vi "CANReadBaseTime.vi"(7 "时间":u32, 8 "日期字符":string) -> (2 "基时间簇":T1)   [LabVIEW 2015]
uses:
  <vilib>/Utility/miscctls.llb/LVDateTimeRec.ctl
  <vilib>/regexp/Match Regular Expression.xnode
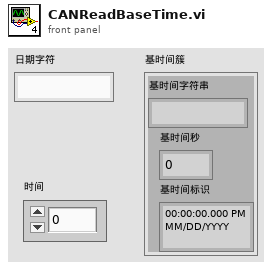
[diagram p1: front panel]
types:
  T1 = cluster{"基时间字符串":string, "基时间秒":dbl, "基时间标识":timestamp}
  T2 = typedef "LVDateTimeRec.ctl" = cluster{"fractional second":dbl, "second":i32, "minute":i32, "hour":i32, "day of month":i32, "month":i32, "year":i32, "day of week":i32, "day of year":i32, "DST":i32}
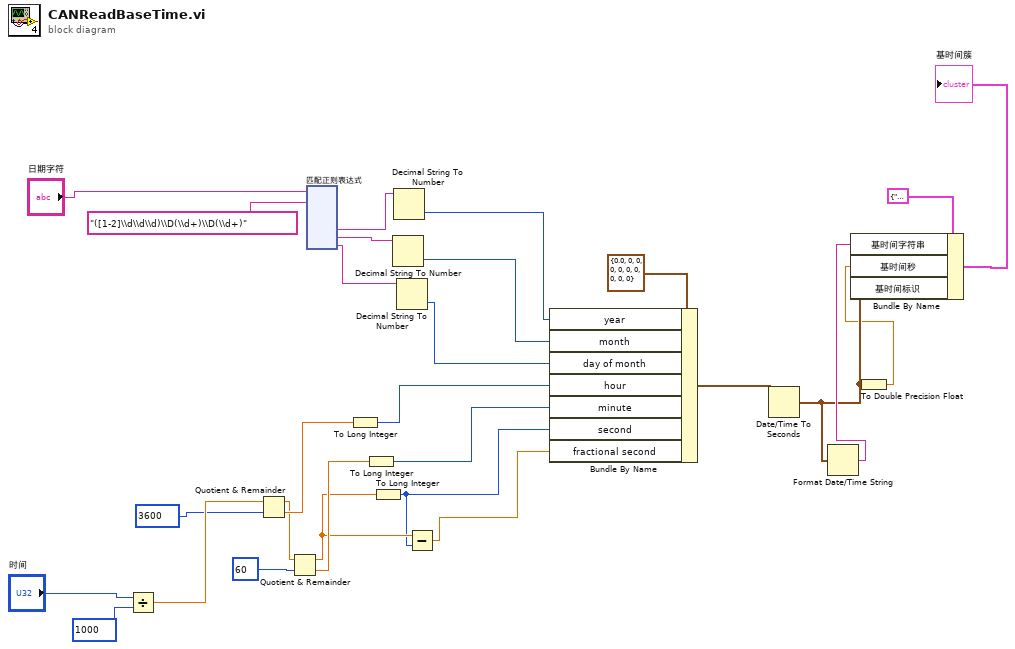
[diagram p0: block diagram]
diagram:
  n1 = Divide(x="时间", y=u32 1000) -> (x/y=w11:dbl)
  n2 = Quotient & Remainder(x=w11, y=3600) -> (x-y*floor(x/y)=w6:dbl, floor(x/y)=w9:dbl)
  n3 = Quotient & Remainder(x=w6, y=60) -> (x-y*floor(x/y)=w3:dbl, floor(x/y)=w5:dbl)
  n4 = xnode "匹配正则表达式"("输入字符串"="日期字符", "正则表达式"="([1-2]\\d\\d\\d)\\D(\\d+)\\D(\\d+)") -> ("子匹配 1"=w20:string, "子匹配 2"=w19:string, "子匹配 3"=w18:string)  [unwired: 4 in, 5 out]
  n5 = To Long Integer(number=w9) -> (32bit integer=w10:i32)
  n6 = To Long Integer(number=w5) -> (32bit integer=w4:i32)
  n7 = To Long Integer(number=w3) -> (32bit integer=w2:i32)
  n8 = Decimal String To Number(string=w19) -> (number=w27:i32)  [unwired: 2 in, 1 out]
  n9 = Decimal String To Number(string=w20) -> (number=w26:i32)  [unwired: 2 in, 1 out]
  n10 = Decimal String To Number(string=w18) -> (number=w28:i32)  [unwired: 2 in, 1 out]
  n11 = Subtract(x=w3, y=w2) -> (x-y=w1:dbl)
  n12 = Bundle By Name(cluster=T2 {"fractional second"=0.0, "second"=0, "minute"=0, "hour"=0, "day of month"=0, "month"=0, "year"=0, "day of week"=0, "day of year"=0, "DST"=0} ("日期时间记录"), "year"=w26, "month"=w27, "day of month"=w28, "hour"=w10, "minute"=w4, "second"=w2, "fractional second"=w1) -> (w15:T2)
  n13 = Date/Time To Seconds(2:w15) -> (0:w24:timestamp)  [unwired: 1 in]
  n14 = Format Date/Time String(seconds (now)=w24) -> (date/time string=w25:string)  [unwired: 2 in]
  n15 = To Double Precision Float(number=w24) -> (double precision float=w23:dbl)
  n16 = Bundle By Name(cluster=T1 {"基时间字符串"="", "基时间秒"=0.0, "基时间标识"=timestamp(0 s since 1904-01-01)} ("基时间簇"), "基时间字符串"=w25, "基时间秒"=w23, "基时间标识"=w24) -> (→"基时间簇":T1)
